vi "level sensor.vi"() -> ()   [LabVIEW 2019]
uses:
  <vilib>/Instr/_visa.llb/VISA Configure Serial Port (Instr).vi
panel:
  in  "Stop Button":bool
  out "Gauge":dbl(knob) scale=0.0..1024.0
  in  "baud rate (9600)":u32=9600
  in  "VISA resource name":refnum<visa-resource-name>
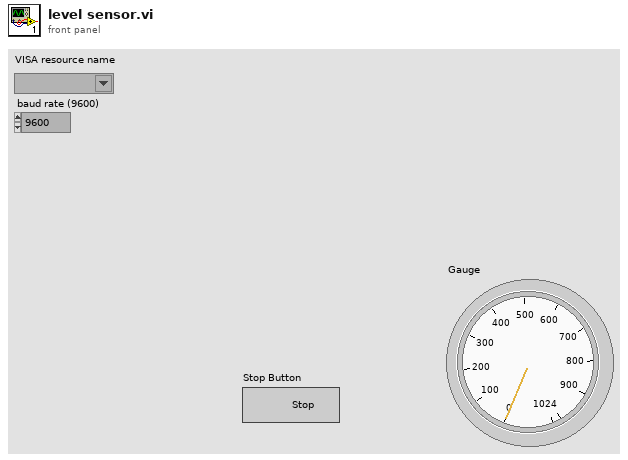
[diagram p1: front panel]
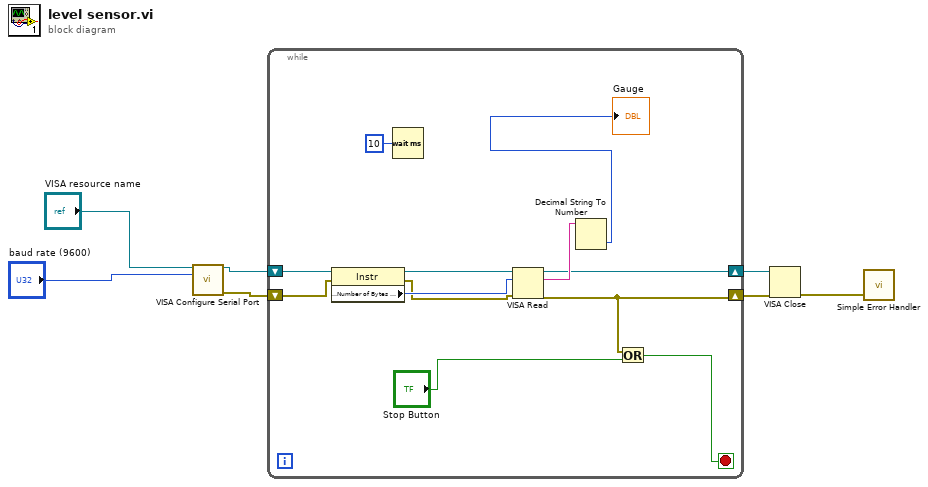
[diagram p0: block diagram]
diagram:
  n1 = call-poly "VISA Configure Serial Port"("VISA resource name"="VISA resource name", "baud rate (9600)"="baud rate (9600)") -> ("VISA resource name out"=w5:refnum<visa-resource-name>, "error out"=w4:errorcluster)  [unwired: 12 in]
  n2 = while {
    shift-right: [w12] -> w3
    shift-left: w5 -> [w19]
    shift-right: [w11] -> w2
    shift-left: w4 -> [w18]
    stop <- w9 stop-if-true
    n3 = property class="Instr"(reference=w19, error in=w18) -> (reference out=w17:refnum<visa-resource-name>, error out=w15:errorcluster, "Serial Settings:Number of Bytes at Serial Port"=w16:u32)
    n4 = Wait (ms)(milliseconds to wait=u32 10) -> ()  [unwired: 1 out]
    n5 = VISA Read(VISA resource name=w17, byte count=w16, error in (no error)=w15) -> (VISA resource name out=w12:refnum<visa-resource-name>, read buffer=w14:string, error out=w11:errorcluster)  [unwired: 1 out]
    n6 = Decimal String To Number(string=w14) -> (number=→"Gauge":i32)  [unwired: 2 in, 1 out]
    n7 = Or(x=w11, y="Stop Button") -> (x .or. y?=w9:bool)
  }
  n8 = VISA Close(VISA resource name=w3, error in (no error)=w2) -> (error out=w1:errorcluster)
  n9 = call <vilib>:"Simple Error Handler.vi"("error in (no error)"=w1) -> ()  [unwired: 4 in, 5 out]
